vi "FG Sensor Buffers Camera SICK.vi"(2 "FG Action (Read)":T2, 3 "Camera SICK Buffer in":T1) -> (1 "Camera SICK Buffer out":T1)   [LabVIEW 2009]
uses:
  Actions for FG's.ctl
  TypeDefs/Sensor TypeDefs/SICK Array.ctl
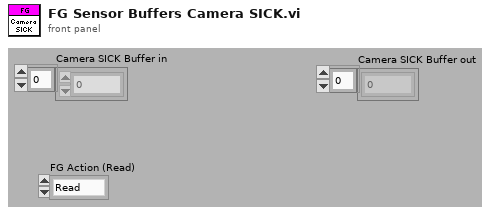
[diagram p1: front panel]
types:
  T1 = typedef "SICK Array.ctl" = u16[]
  T2 = typedef "Actions for FG's.ctl" = enum16{"Read", "Write"}
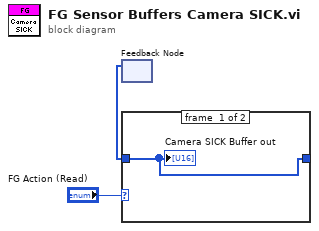
[diagram p0: block diagram]
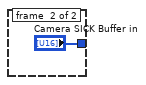
[diagram p2: hidden frame]
diagram:
  n1 = feedback #1() -> (w1:T1)  [unwired: 1 in]
  n2 = case shown="\"Read\", Default" "FG Action (Read)" {
    tunnel: w1 -> [w4 _]
    tunnel: [w4 "Camera SICK Buffer in"] -> w2
    frame #0 {
      "Camera SICK Buffer out" <- w4
    }
    frame #1 {
    }
  }
